vi "Write Message Type.lvclass.vi"(8 "error in (no error)":errorcluster, 10 "Message Type.lvclass":refnum<class "Message Type.lvclass">, 11 "User Sender in":refnum<class "User Sender.lvclass">) -> (0 "error out":errorcluster, 3 "User Sender out":refnum<class "User Sender.lvclass">)   [LabVIEW 2023, in "User Sender.lvclass"]
uses:
  User Sender.lvclass
  User Sender.lvclass/User Sender.ctl
  Message Type/Message Type.lvclass
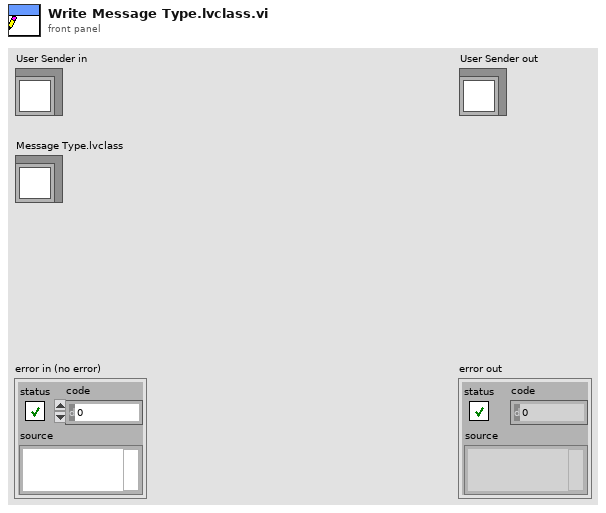
[diagram p1: front panel]
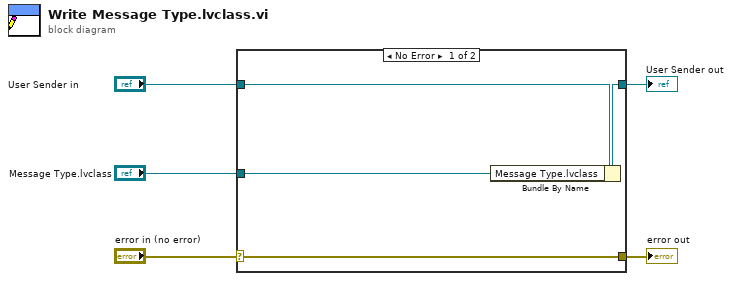
[diagram p0: block diagram]
diagram:
  n1 = case shown="No Error" "error in (no error)" {
    selector: "error in (no error)" -> [w9 w10]
    tunnel: [w9 w10] -> w4
    tunnel: [w7 w11] -> w2
    tunnel: "User Sender in" -> [w8 w11]
    tunnel: "Message Type.lvclass" -> [w6 _]
    frame No Error {
      n2 = Bundle By Name(cluster=w8, "Message Type.lvclass"=w6) -> (w7:refnum<class "User Sender.lvclass">)
    }
    frame Error {
    }
  }
  "error out" <- w4
  "User Sender out" <- w2
